vi "Custom label Print.vi"() -> ()   [LabVIEW 2018]
panel:
  out "EOL Stations":string
  out "OEM":string
  in  "停止":bool
  out "error out":errorcluster
  out "Ser nr":string
  out "IRS nr":string
  in  "簇":T1
  # "标签预览"
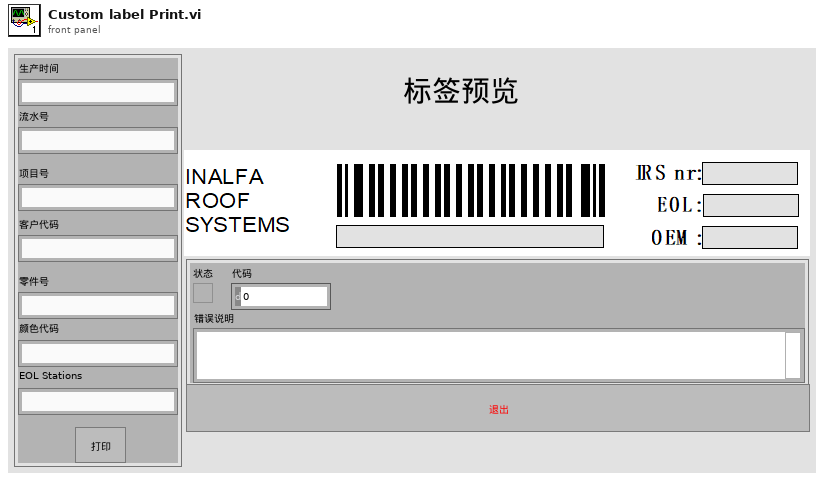
[diagram p1: front panel]
types:
  T1 = cluster{"生产时间":string, "流水号":string, "项目号":string, "客户代码":string, "零件号":string, "打印":bool, "颜色代码":string, "EOL Stations":string}
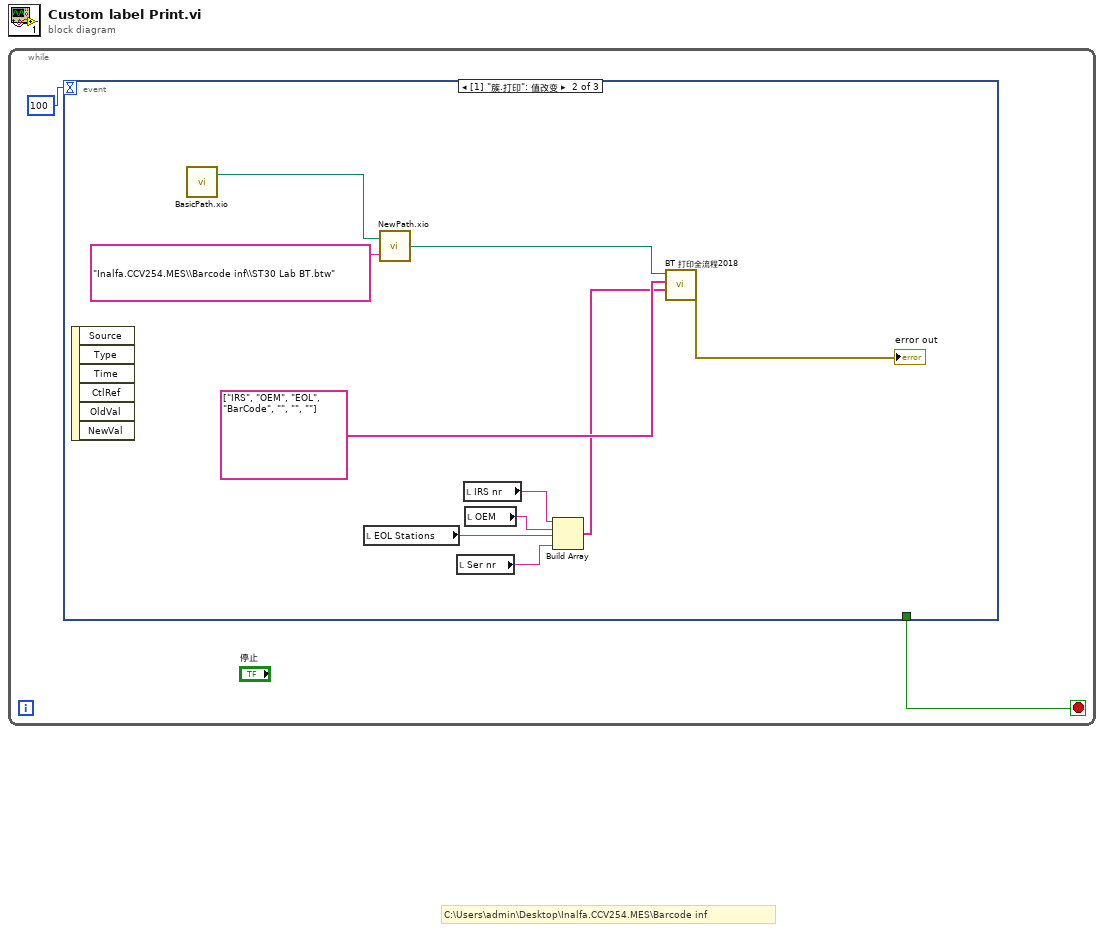
[diagram p0: block diagram]
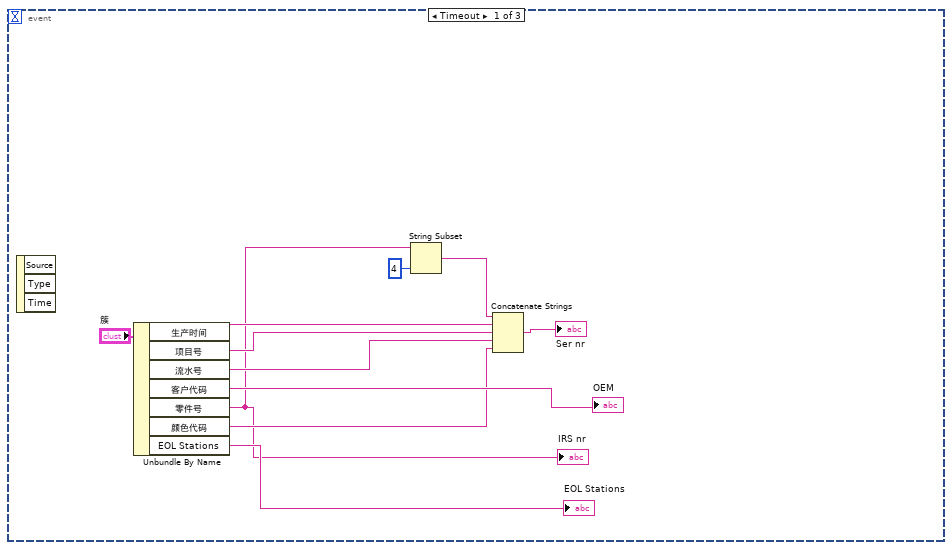
[diagram p2: hidden frame]
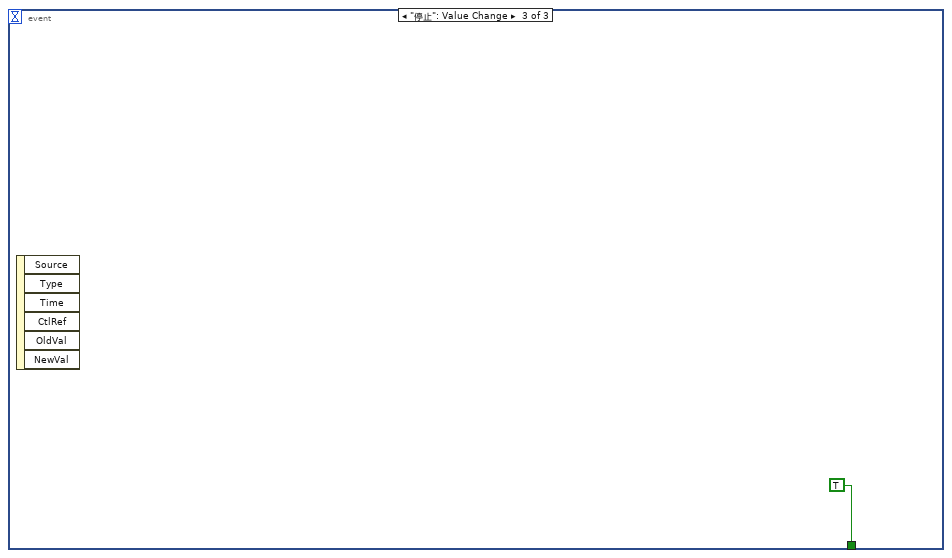
[diagram p3: hidden frame]
diagram:
  # "C:\\Users\\admin\\Desktop\\Inalfa.CCV254.MES\\Barcode inf"
  n1 = while {
    stop <- w2 stop-if-true
    n2 = event shown="[1] \"簇.打印\": 值改变" {
      selector: _ -> [_ _ _]
      dyn-events: _ -> [_ _ _]
      timeout: 100 -> [_ _ _]
      tunnel: [_ _ TRUE] -> w2
      event Timeout {
        n3 = event-data() -> ()  [unwired: 1 in, 3 out]
        n4 = Unbundle By Name("簇") -> ("生产时间"=w12:string, "项目号"=w9:string, "流水号"=w8:string, "客户代码"=→"OEM":string, "零件号"=w5:string, "颜色代码"=w7:string, "EOL Stations"=→"EOL Stations":string)
        "IRS nr" <- w5
        n5 = String Subset(string=w5, length (rest)=4 ("长度（剩余）")) -> (substring=w3:string)  [unwired: 1 in]
        n6 = Concatenate Strings(w3, w12, w9, w8, w7) -> (→"Ser nr":string)
      }
      event "簇.打印": Value Change {
        n7 = event-data() -> ()  [unwired: 1 in, 6 out]
        n8 = call "BasicPath.xio.vi"() -> ("stripped path"=w19:path)  [unwired: 1 in, 1 out]
        n9 = local read "EOL Stations"() -> (w21:string)
        n10 = call "NewPath.xio.vi"("Append path"="Inalfa.CCV254.MES\\Barcode inf\\ST30 Lab BT.btw", "Basic path"=w19) -> ("New path"=w17:path)
        n11 = local read "Ser nr"() -> (w20:string)
        n12 = local read "IRS nr"() -> (w22:string)
        n13 = local read "OEM"() -> (w23:string)
        n14 = Build Array(w22, w23, w21, w20) -> (w15:string[])
        n15 = call "BT 打印全流程2018.vi"("文件路径"=w17, "BT 具名数据源名称"=string[] ["IRS", "OEM", "EOL", "BarCode", "", "", ""], "输入内容"=w15) -> ("error out"=→"error out":errorcluster)  [unwired: 7 in]
      }
      event "停止": Value Change {
        n16 = event-data() -> ()  [unwired: 1 in, 6 out]
      }
    }
  }
